vi "Append VI Description to Report (string).vi"(0 "report in":refnum<class "NI_report.lvclass">, 5 "VI":string, 11 "error in (no error)":errorcluster, 12 "MS Office parameters":T1) -> (4 "report out":refnum<class "NI_report.lvclass">, 6 "VI name out":string, 8 "start out (Word)":i32, 10 "end out (Word)":i32, 15 "error out":errorcluster)   [LabVIEW 2020, in "NI_ReportGenerationCore.lvlib"]
doc: "Appends the description of the VI you specify in <B>VI</B> to a report. Wire data to the <B>VI</B> input to determine the polymorphic instance to use or manually select the instance."
uses:
  <vilib>/Utility/NIReport.llb/NI_ReportGenerationCore.lvlib
  <vilib>/Utility/NIReport.llb/NI_report.lvclass
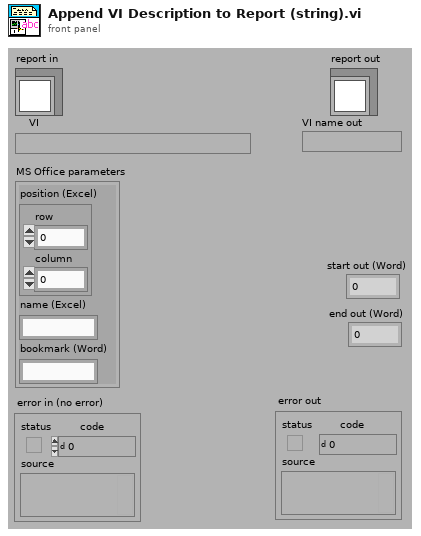
[diagram p1: front panel]
types:
  T1 = cluster{"position (Excel)":cluster{"row":i32, "column":i32}, "name (Excel)":string, "bookmark (Word)":string}
  T2 = enum32{"invalid app kind", "Development System", "Run Time System", "Student Edition", "Embedded LabVIEW", "Evaluation", "Custom"}
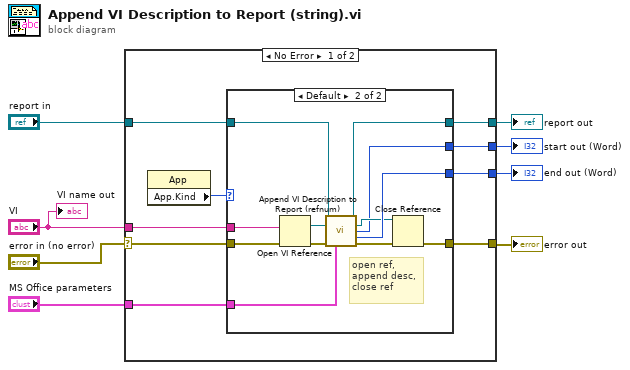
[diagram p0: block diagram]
diagram:
  n1 = case shown="No Error" "error in (no error)" {
    selector: "error in (no error)" -> [w16 w32]
    tunnel: [w14 w32] -> w7
    tunnel: [w12 w33] -> w5
    tunnel: "report in" -> [w11 w33]
    tunnel: "VI" -> [w17 _]
    tunnel: "MS Office parameters" -> [w15 _]
    tunnel: [w10 _] -> w2
    tunnel: [w13 _] -> w1
    frame No Error {
      n2 = property class="App"() -> ("App.Kind"=w9:T2)  [unwired: 2 in, 2 out]
      n3 = case shown="Default" w9 {
        tunnel: w17 -> [_ w31]
        tunnel: w16 -> [w18 w30]
        tunnel: w15 -> [_ w27]
        tunnel: [w18 w25] -> w14
        tunnel: [_ w24] -> w13
        tunnel: [w19 w23] -> w12
        tunnel: w11 -> [w19 w22]
        tunnel: [_ w20] -> w10
        frame "Run Time System" {
          # "Do not try to append\nif running in an\nexecutable"
        }
        frame Default {
          # "open ref,\nappend desc,\nclose ref"
          n4 = Open VI Reference(vi path=w31, error in (no error)=w30) -> (vi reference=w29:refnum<vi>, error out=w28:errorcluster)  [unwired: 4 in]
          n5 = call <vilib>:"Append VI Description to Report (refnum).vi"("report in"=w22, "VI"=w29, "error in (no error)"=w28, "MS Office parameters"=w27) -> ("report out"=w23:refnum<class "NI_report.lvclass">, "VI out"=w21:refnum<vi>, "start out (Word)"=w20:i32, "end out (Word)"=w24:i32, "error out"=w26:errorcluster)  [unwired: 7 in]
          n6 = Close Reference(reference=w21, error in (no error)=w26) -> (error out=w25:errorcluster)
        }
      }
    }
    frame Error {
    }
  }
  "error out" <- w7
  "report out" <- w5
  "start out (Word)" <- w2
  "end out (Word)" <- w1
  "VI name out" <- "VI"
